vi "Chk Value(SubVI).vi"(10 "Password":string, 11 "User Name":string) -> (3 "Boolean":bool)   [LabVIEW 2024]
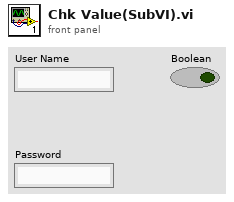
[diagram p1: front panel]
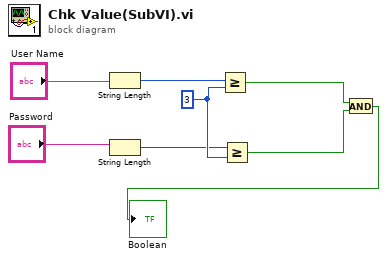
[diagram p0: block diagram]
diagram:
  w5 = 3 ("y")
  n1 = String Length(string="User Name") -> (length=w3:i32)
  n2 = String Length(string="Password") -> (length=w4:i32)
  n3 = Greater Or Equal?(x=w3, y=w5) -> (x >= y?=w6:bool)
  n4 = Greater Or Equal?(x=w4, y=w5) -> (x >= y?=w7:bool)
  n5 = And(x=w6, y=w7) -> (x .and. y?=→"Boolean":bool)
